vi "frontp_get_hardware_caller_queue.vi"(8 "error in (no error)":errorcluster, 10 "hardware":T1, 11 "front_panel in":refnum<class "front_panel.lvclass">) -> (0 "error out":errorcluster, 2 "Nested Actor's Enqueuer":refnum<class "Message Enqueuer.lvclass">, 3 "front_panel out":refnum<class "front_panel.lvclass">)   [LabVIEW 2015, in "front_panel.lvclass"]
uses:
  front_panel.lvclass
  hardware_caller_queue_numbers.ctl
  <vilib>/ActorFramework/Message Enqueuer/Message Enqueuer.lvclass
  front_panel.lvclass/front_panel.ctl
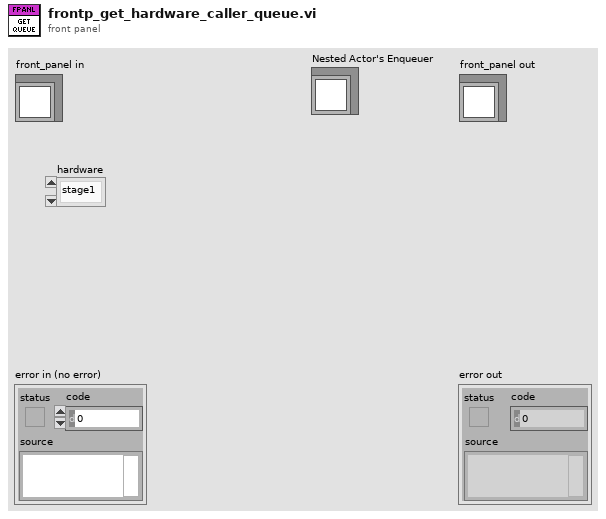
[diagram p1: front panel]
types:
  T1 = typedef "hardware_caller_queue_numbers.ctl" = enum16{"stage1", "stage2", "experiment", "detector"}
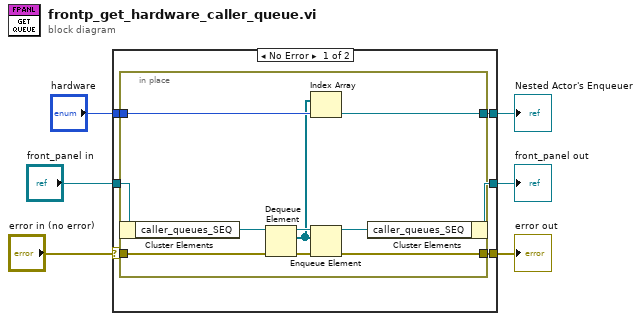
[diagram p0: block diagram]
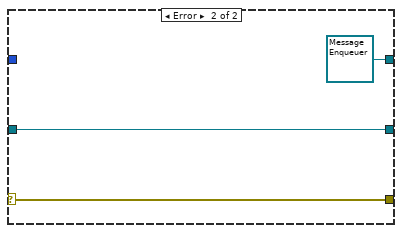
[diagram p2: hidden frame]
diagram:
  n1 = case shown="No Error" "error in (no error)" {
    selector: "error in (no error)" -> [w11 w24]
    tunnel: [w8 w24] -> w5
    tunnel: [w7 w23] -> w3
    tunnel: "front_panel in" -> [w12 w23]
    tunnel: "hardware" -> [w10 _]
    tunnel: [w9 refnum<class "Message Enqueuer.lvclass"> refnum ("Nested Actor's Enqueuer")] -> w1
    frame No Error {
      n2 = in-place {
        in-place-border: w11 -> [w20]
        in-place-border: w10 -> [w19]
        in-place-border: [w18] -> w9
        in-place-border: [w13] -> w8
        n3 = in-place-cluster #1(w12) -> ("caller_queues_SEQ"=w21:refnum<queue>)
        n4 = Dequeue Element(queue=w21, error in (no error)=w20) -> (queue out=w16:refnum<queue>, element=w15:refnum<class "Message Enqueuer.lvclass">[], error out=w17:errorcluster)  [unwired: 1 in, 1 out]
        n5 = Index Array(array=w15, index=w19) -> (element=w18:refnum<class "Message Enqueuer.lvclass">)
        n6 = Enqueue Element(queue=w16, element=w15, error in (no error)=w17) -> (queue out=w14:refnum<queue>, error out=w13:errorcluster)  [unwired: 1 in, 1 out]
        n7 = in-place-cluster #1("caller_queues_SEQ"=w14) -> (w7:refnum<class "front_panel.lvclass">)
      }
    }
    frame Error {
    }
  }
  "error out" <- w5
  "front_panel out" <- w3
  "Nested Actor's Enqueuer" <- w1
